vi "CheckState.vi"(10 "Current state in":string, 11 "Last state":string) -> (3 "Update?":bool)   [LabVIEW 2020]
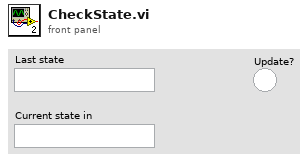
[diagram p1: front panel]
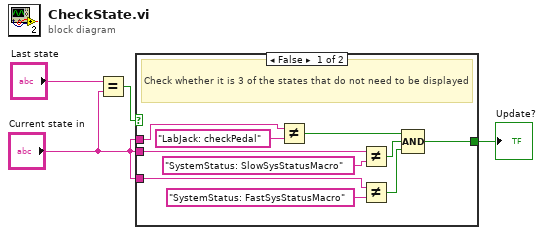
[diagram p0: block diagram]
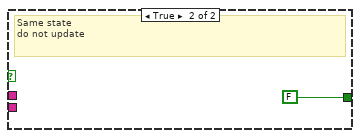
[diagram p2: hidden frame]
diagram:
  n1 = Equal?(x="Last state", y="Current state in") -> (x = y?=w3:bool)
  n2 = case shown="False" w3 {
    tunnel: [w5 FALSE] -> w2
    tunnel: "Current state in" -> [w10 _]
    tunnel: "Current state in" -> [w8 _]
    tunnel: "Current state in" -> [w6 _]
    frame False {
      # "Check whether it is 3 of the states that do not need to be displayed"
      n3 = Not Equal?(x=w6, y="LabJack: checkPedal") -> (x != y?=w14:bool)
      n4 = Not Equal?(x=w8, y="SystemStatus: SlowSysStatusMacro") -> (x != y?=w13:bool)
      n5 = Not Equal?(x=w10, y="SystemStatus: FastSysStatusMacro") -> (x != y?=w12:bool)
      n6 = Compound Arithmetic op=AND(w14, w13, w12) -> (w5:bool)
    }
    frame True {
      # "Same state\ndo not update"
    }
  }
  "Update?" <- w2
